vi "StripRelativePath.vi"(0 "URL":path, 5 "Levels To Strip":i32) -> (4 "Stripped URL":path)   [LabVIEW 2017]
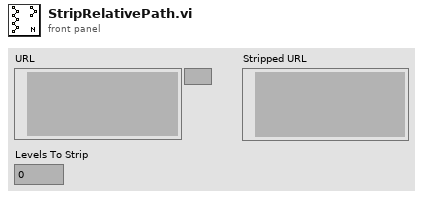
[diagram p1: front panel]
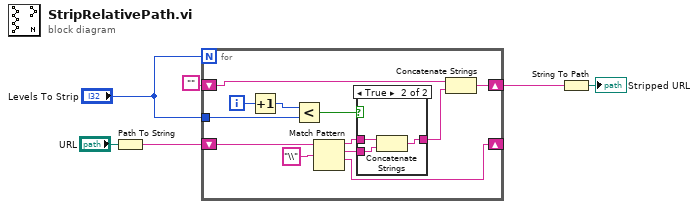
[diagram p0: block diagram]
diagram:
  n1 = Path To String(path="URL") -> (string=w6:string)
  n2 = for {
    N: "Levels To Strip" -> [_]
    shift-right: [w14] -> _
    shift-left: w6 -> [w17]
    tunnel: "Levels To Strip" -> [w11]
    shift-right: [w8] -> w2
    shift-left: "" -> [w7]
    i -> [w12]
    n3 = Increment(x=w12) -> (x+1=w10:i32)
    n4 = Less?(x=w10, y=w11) -> (x < y?=w9:bool)
    n5 = Match Pattern(string=w17, regular expression="\\" ("search string/char (-)")) -> (before substring=w16:string, match substring=w13:string, after substring=w14:string)  [unwired: 1 in, 1 out]
    n6 = case shown="True" w9 {
      tunnel: w16 -> [w19 w22]
      tunnel: [w19 w21] -> w15
      tunnel: w13 -> [_ w20]
      frame False {
      }
      frame True {
        n7 = Concatenate Strings(w22, w20) -> (w21:string)
      }
    }
    n8 = Concatenate Strings(w7, w15) -> (w8:string)
  }
  n9 = String To Path(string=w2) -> (path=→"Stripped URL":path)
